vi "save.vi"(5 "log?":bool, 8 "queue in":refnum<queue>, 11 "Qube":refnum<class "System.lvclass">) -> (3 "Qube":refnum<class "System.lvclass">)   [LabVIEW 2021, in "System.lvclass"]
uses:
  System.lvclass
  System.lvclass/System.ctl
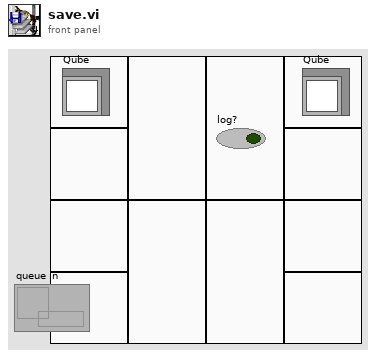
[diagram p1: front panel]
types:
  T1 = enum16{"big-endian, network order", "native, host order", "little-endian"}
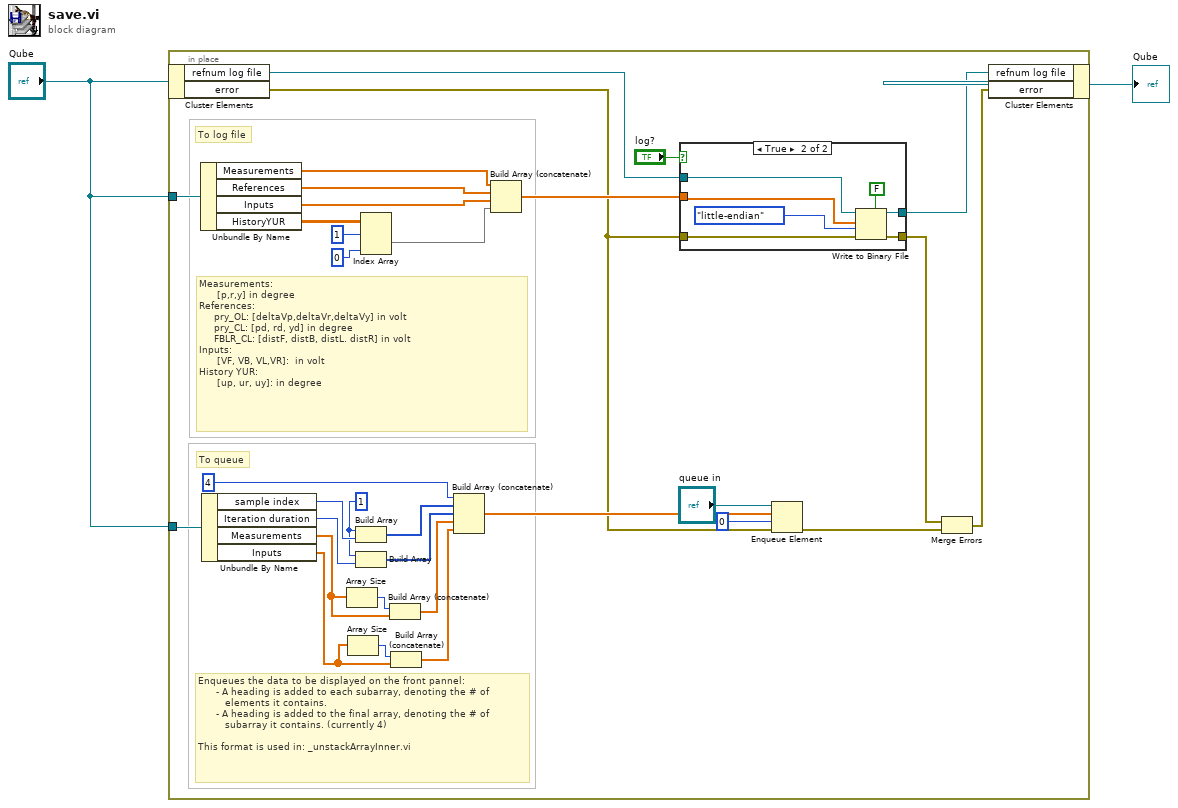
[diagram p0: block diagram]
diagram:
  n1 = in-place {
    in-place-border: "Qube" -> [w29]
    in-place-border: "Qube" -> [w27]
    w11 = u32 1 ("element")
    # "Enqueues the data to be displayed on the front pannel:\n      - A heading is added to each subarray, denoting the # of\n         elements it contains. \n      - A heading is added to the final array, denoting the # of\n         subarray it contains. (currently 4)\n\nThis format is used in: _unstackArrayInner.vi"
    # "To queue"
    # "To log file"
    # "Measurements: \n      [p,r,y] in degree\nReferences: \n     pry_OL: [deltaVp,deltaVr,deltaVy] in volt\n     pry_CL: [pd, rd, yd] in degree\n     FBLR_CL: [distF, distB, distL. distR] in volt\nInputs:\n      [VF, VB, VL,VR]:  in volt\nHistory YUR:\n      [up, ur, uy]: in degree"
    n2 = in-place-cluster #1("Qube") -> ("refnum log file"=w26:refnum<file>, "error"=w3:errorcluster)
    n3 = Unbundle By Name(w29) -> ("Measurements"=w7:dbl[], "References"=w6:dbl[], "Inputs"=w5:dbl[], "HistoryYUR"=w10:dbl[][][])
    n4 = Unbundle By Name(w27) -> ("sample index"=w23:u32, "Iteration duration"=w22:u32, "Measurements"=w13:dbl[], "Inputs"=w17:dbl[])
    n5 = Array Size(array=w13) -> (size(s)=w19:i32)
    n6 = Array Size(array=w17) -> (size(s)=w18:i32)
    n7 = Build Array(w11, w23) -> (w21:u32[])
    n8 = Build Array(w11, w22) -> (w20:u32[])
    n9 = Index Array(array=w10, index (dim 0)=1 ("index (page)"), index (dim 2)=0 ("disabled index (col)")) -> (element=w4:dbl[])  [unwired: 1 in]
    n10 = Build Array (concatenate)(w19, w13) -> (w16:dbl[])
    n11 = Build Array (concatenate)(w18, w17) -> (w15:dbl[])
    n12 = Build Array (concatenate)(u32 4 ("element"), w21, w20, w16, w15) -> (w14:dbl[])
    n13 = Build Array (concatenate)(w7, w6, w5, w4) -> (w28:dbl[])
    n14 = case shown="True" "log?" {
      tunnel: w3 -> [w35 w42]
      tunnel: w28 -> [_ w40]
      tunnel: w26 -> [w36 w39]
      tunnel: [w35 w38] -> w31
      tunnel: [w36 w37] -> w25
      frame False {
      }
      frame True {
        n15 = Write to Binary File(file (use dialog)=w39, data=w40, error in=w42, 5:FALSE ("prepend array or string size? (T)"), 9:T1."little-endian" ("byte order (0:big-endian, network order)")) -> (refnum out=w37:refnum<file>, error out=w38:errorcluster)  [unwired: 1 in, 1 out]
      }
    }
    n16 = Enqueue Element(queue="queue in", element=w14, timeout in ms (-1)=0, error in (no error)=w3) -> (error out=w32:errorcluster)  [unwired: 2 out]
    n17 = Merge Errors(w31, w32) -> (w24:errorcluster)
    n18 = in-place-cluster #1("refnum log file"=w25, "error"=w24) -> (→"Qube":refnum<class "System.lvclass">)
  }
